vi "Queue Manager.vi"(5 "Queue Name":T3, 6 "timeout in ms (-1)":i32=-1, 7 "Action":T2=enum."Enqueue", 8 "Error In":errorcluster, 11 "Message Packet Array":T1[](array[typedef])) -> (0 "Error Out":errorcluster, 1 "Empty?":bool, 2 "# elements in queue":i32, 3 "Message Packet [Out]":T1, 4 "elements":T1[](array[typedef]))   [LabVIEW 2018]
uses:
  Controls/QueueNames.ctl
  Controls/Queue Manager Actions.ctl
  Controls/MessagePacket.ctl
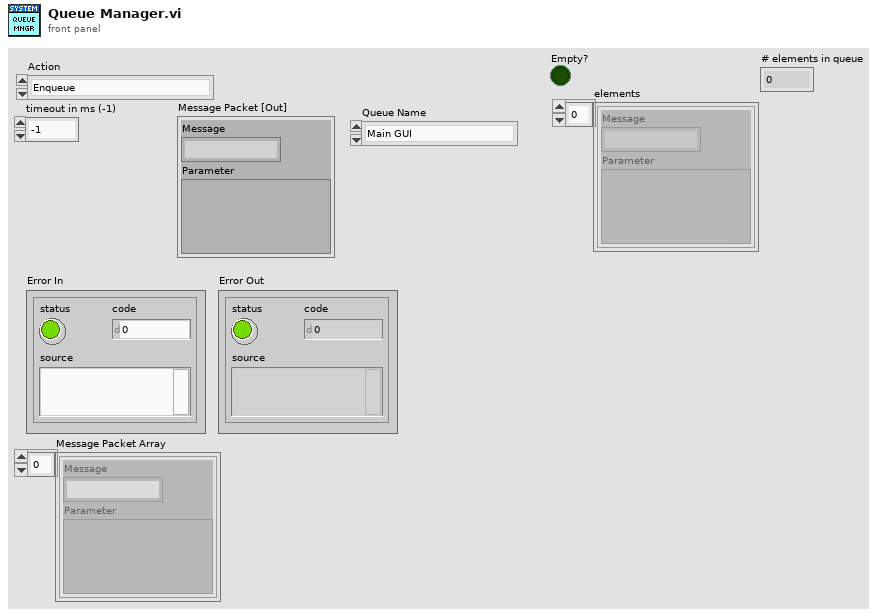
[diagram p1: front panel]
types:
  T1 = typedef "MessagePacket.ctl" = cluster{"Message":string, "Parameter":variant}
  T2 = typedef "Queue Manager Actions.ctl" = enum16{"Init", "Enqueue", "Enqueue All", "Preview Queue", "Dequeue", "Get Status", "Flush Queue", "Flush All Queues", "Release All Queues", "Release Queue", "Enqueue at Opposite End"}
  T3 = typedef "QueueNames.ctl" = enum16{"Main GUI", "Main Scan Processor", "Main Display Processing", "Main Processing", "Main Saving", "Main Display", "Main Table Stage GUI", "Main Table Stage Proc.", "Scan Engine", "Vibratome GUI", "Vibratome Processor", "Slice Engine"}
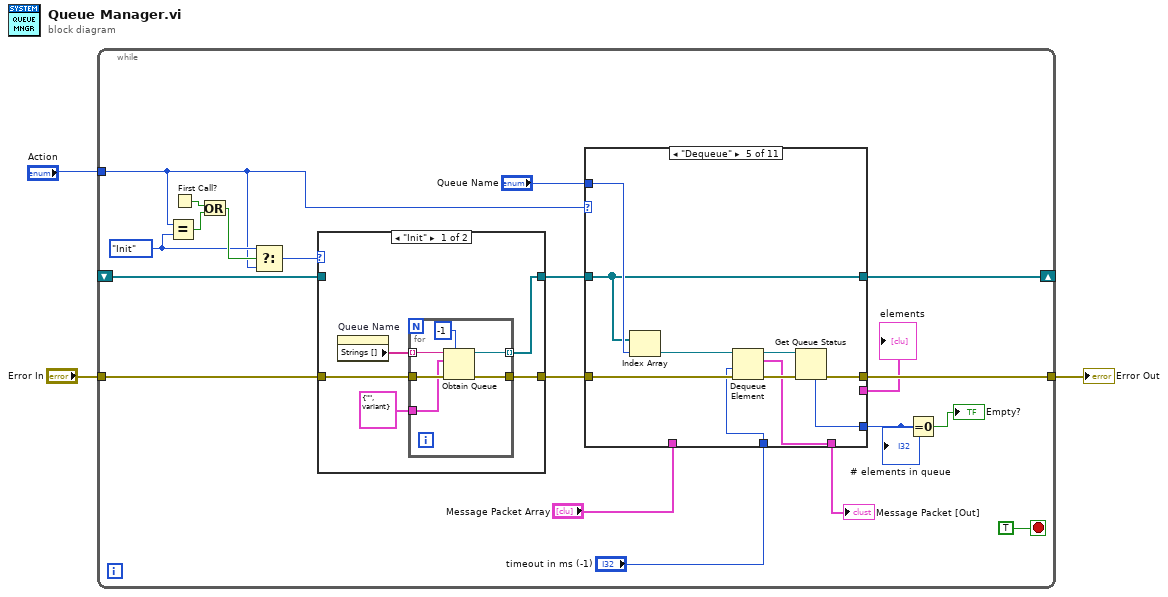
[diagram p0: block diagram]
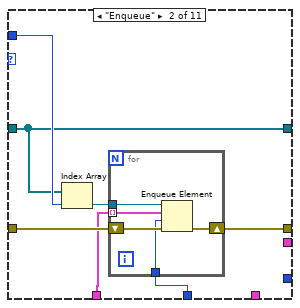
[diagram p3: hidden frame]
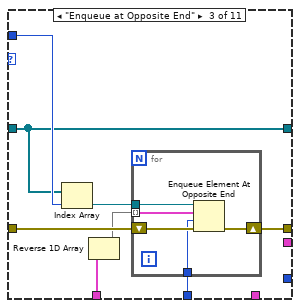
[diagram p4: hidden frame]
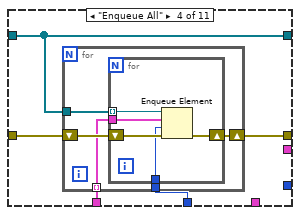
[diagram p5: hidden frame]
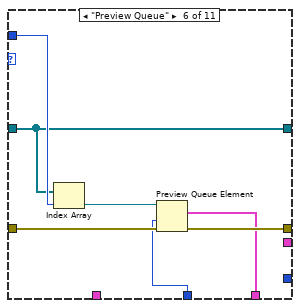
[diagram p6: hidden frame]
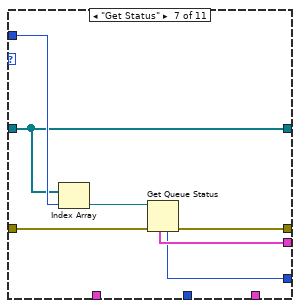
[diagram p7: hidden frame]
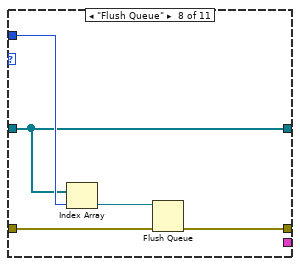
[diagram p8: hidden frame]
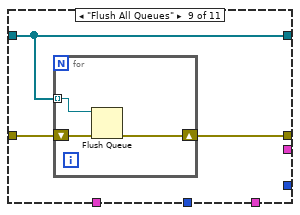
[diagram p9: hidden frame]
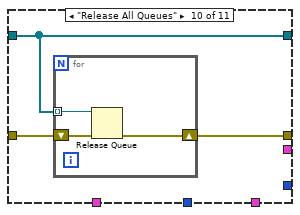
[diagram p10: hidden frame]
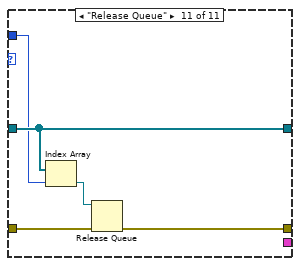
[diagram p11: hidden frame]
diagram:
  n1 = while {
    tunnel: "Action" -> [w8]
    tunnel: "Error In" -> [w18]
    tunnel: [w17] -> w1
    shift-right: [w10] -> _
    shift-left: _ -> [w9]
    stop <- TRUE stop-if-true
    w20 = Queue_Manager_Actions."Init"
    n2 = Equal?(x=w8, y=w20) -> (x = y?=w22:bool)
    n3 = First Call?() -> (First Call?: T/F=w23:bool)
    n4 = Or(x=w23, y=w22) -> (x .or. y?=w21:bool)
    n5 = Select(t=w20, s=w21, f=w8) -> (s? t:f=w19:T2)
    n6 = case shown="\"Init\"" w19 {
      tunnel: [w115 w123] -> w14
      tunnel: w18 -> [w114 w124]
      tunnel: [w113 w124] -> w16
      tunnel: w9 -> [_ w123]
      frame "Init" {
        n7 = property on="Queue Name" class="Enum (strict)"() -> ("Strings []"=w116:string[])  [unwired: 2 in, 2 out]
        n8 = for {
          tunnel: w116 -> [w122] mode=indexing
          tunnel: [w121] -> w115 mode=indexing
          tunnel: w114 -> [w120]
          tunnel: [w119] -> w113
          tunnel: T1 {"Message"="", "Parameter"=variant} ("Message Packet") -> [w118]
          n9 = Obtain Queue(max queue size (-1, unlimited)=-1, name (unnamed)=w122, element data type=w118, error in (no error)=w120) -> (queue out=w121:refnum<queue>, error out=w119:errorcluster)  [unwired: 1 in, 1 out]
        }
      }
      frame "Enqueue", Default {
      }
    }
    n10 = case shown="\"Dequeue\"" w8 {
      tunnel: w14 -> [w24 w27 w40 w52 w70 w77 w85 w90 w95 w101 w109]
      tunnel: [w25 w31 w44 w54 w68 w81 w88 w91 w96 w102 w110] -> w17
      tunnel: w16 -> [w25 w32 w45 w55 w75 w82 w89 w94 w97 w103 w111]
      tunnel: "Queue Name" -> [_ w30 w43 _ w73 w80 w87 w93 _ _ w108]
      tunnel: "Message Packet Array" -> [_ w28 w41 w53 _ _ _ _ _ _ _]
      tunnel: [_ _ _ _ w71 w78 _ _ _ _ _] -> w13
      tunnel: [w24 w27 w40 w52 w70 w77 w85 w90 w95 w101 w109] -> w10
      tunnel: "timeout in ms (-1)" -> [_ w26 w38 w51 w69 w76 _ _ _ _ _]
      tunnel: [_ _ _ _ _ _ w84 _ _ _ _] -> w6
      tunnel: [_ _ _ _ w66 _ w83 _ _ _ _] -> w5
      frame "Init", Default {
      }
      frame "Enqueue" {
        n11 = Index Array(array=w27, index=w30) -> (element=w29:refnum<queue>)
        n12 = for {
          tunnel: w29 -> [w35]
          tunnel: w28 -> [w34] mode=indexing
          shift-right: [w36] -> w31
          shift-left: w32 -> [w37]
          tunnel: w26 -> [w33]
          n13 = Enqueue Element(queue=w35, element=w34, timeout in ms (-1)=w33, error in (no error)=w37) -> (error out=w36:errorcluster)  [unwired: 2 out]
        }
      }
      frame "Enqueue at Opposite End" {
        n14 = Index Array(array=w40, index=w43) -> (element=w42:refnum<queue>)
        n15 = Reverse 1D Array(array=w41) -> (reversed array=w39:T1[])
        n16 = for {
          tunnel: w42 -> [w48]
          tunnel: w39 -> [w47] mode=indexing
          shift-right: [w49] -> w44
          shift-left: w45 -> [w50]
          tunnel: w38 -> [w46]
          n17 = Enqueue Element At Opposite End(queue=w48, element=w47, timeout in ms (-1)=w46, error in (no error)=w50) -> (error out=w49:errorcluster)  [unwired: 2 out]
        }
      }
      frame "Enqueue All" {
        n18 = for {
          tunnel: w53 -> [w58] mode=indexing
          shift-right: [w59] -> w54
          shift-left: w55 -> [w60]
          tunnel: w52 -> [w57]
          tunnel: w51 -> [w56]
          n19 = for {
            tunnel: w57 -> [w63] mode=indexing
            tunnel: w58 -> [w62]
            shift-right: [w64] -> w59
            shift-left: w60 -> [w65]
            tunnel: w56 -> [w61]
            n20 = Enqueue Element(queue=w63, element=w62, timeout in ms (-1)=w61, error in (no error)=w65) -> (error out=w64:errorcluster)  [unwired: 2 out]
          }
        }
      }
      frame "Dequeue" {
        n21 = Index Array(array=w70, index=w73) -> (element=w72:refnum<queue>)
        n22 = Dequeue Element(queue=w72, timeout in ms (-1)=w69, error in (no error)=w75) -> (queue out=w67:refnum<queue>, element=w71:T1, error out=w74:errorcluster)  [unwired: 1 out]
        n23 = Get Queue Status(queue=w67, error in (no error)=w74) -> (error out=w68:errorcluster, # elements in queue=w66:i32)  [unwired: 1 in, 6 out]
      }
      frame "Preview Queue" {
        n24 = Index Array(array=w77, index=w80) -> (element=w79:refnum<queue>)
        n25 = Preview Queue Element(queue=w79, timeout in ms (-1)=w76, error in (no error)=w82) -> (element=w78:T1, error out=w81:errorcluster)  [unwired: 2 out]
      }
      frame "Get Status" {
        n26 = Index Array(array=w85, index=w87) -> (element=w86:refnum<queue>)
        n27 = Get Queue Status(queue=w86, error in (no error)=w89) -> (error out=w88:errorcluster, # elements in queue=w83:i32, elements=w84:T1[])  [unwired: 1 in, 5 out]
      }
      frame "Flush Queue" {
        n28 = Index Array(array=w90, index=w93) -> (element=w92:refnum<queue>)
        n29 = Flush Queue(queue=w92, error in (no error)=w94) -> (error out=w91:errorcluster)  [unwired: 2 out]
      }
      frame "Flush All Queues" {
        n30 = for {
          shift-right: [w99] -> w96
          shift-left: w97 -> [w100]
          tunnel: w95 -> [w98] mode=indexing
          n31 = Flush Queue(queue=w98, error in (no error)=w100) -> (error out=w99:errorcluster)  [unwired: 2 out]
        }
      }
      frame "Release All Queues" {
        n32 = for {
          shift-right: [w105] -> w102
          shift-left: w103 -> [w106]
          tunnel: w101 -> [w104] mode=indexing
          n33 = Release Queue(queue=w104, error in (no error)=w106) -> (error out=w105:errorcluster)  [unwired: 1 in, 2 out]
        }
      }
      frame "Release Queue" {
        n34 = Index Array(array=w109, index=w108) -> (element=w107:refnum<queue>)
        n35 = Release Queue(queue=w107, error in (no error)=w111) -> (error out=w110:errorcluster)  [unwired: 1 in, 2 out]
      }
    }
    "Message Packet [Out]" <- w13
    "elements" <- w6
    "# elements in queue" <- w5
    n36 = Equal To 0?(x=w5) -> (x = 0?=→"Empty?":bool)
  }
  "Error Out" <- w1
